vi "Window_plot.vi"() -> ()   [LabVIEW 2022 SP3]
doc: "This window has the capability to visualize and analyze the graphs of the stored signals from the Main_menu."
uses:
  <vilib>/Waveform/WDTOps.llb/WDT Get Waveform Subset DBL.vi
panel:
  in  "Slide Offset":i32(slide) scale=0.0..10.0
  in  "Select offset":string(combo)
  out "Waveform Graph":waveform(dbl)[](graph) caption="Waveform Graph 2"
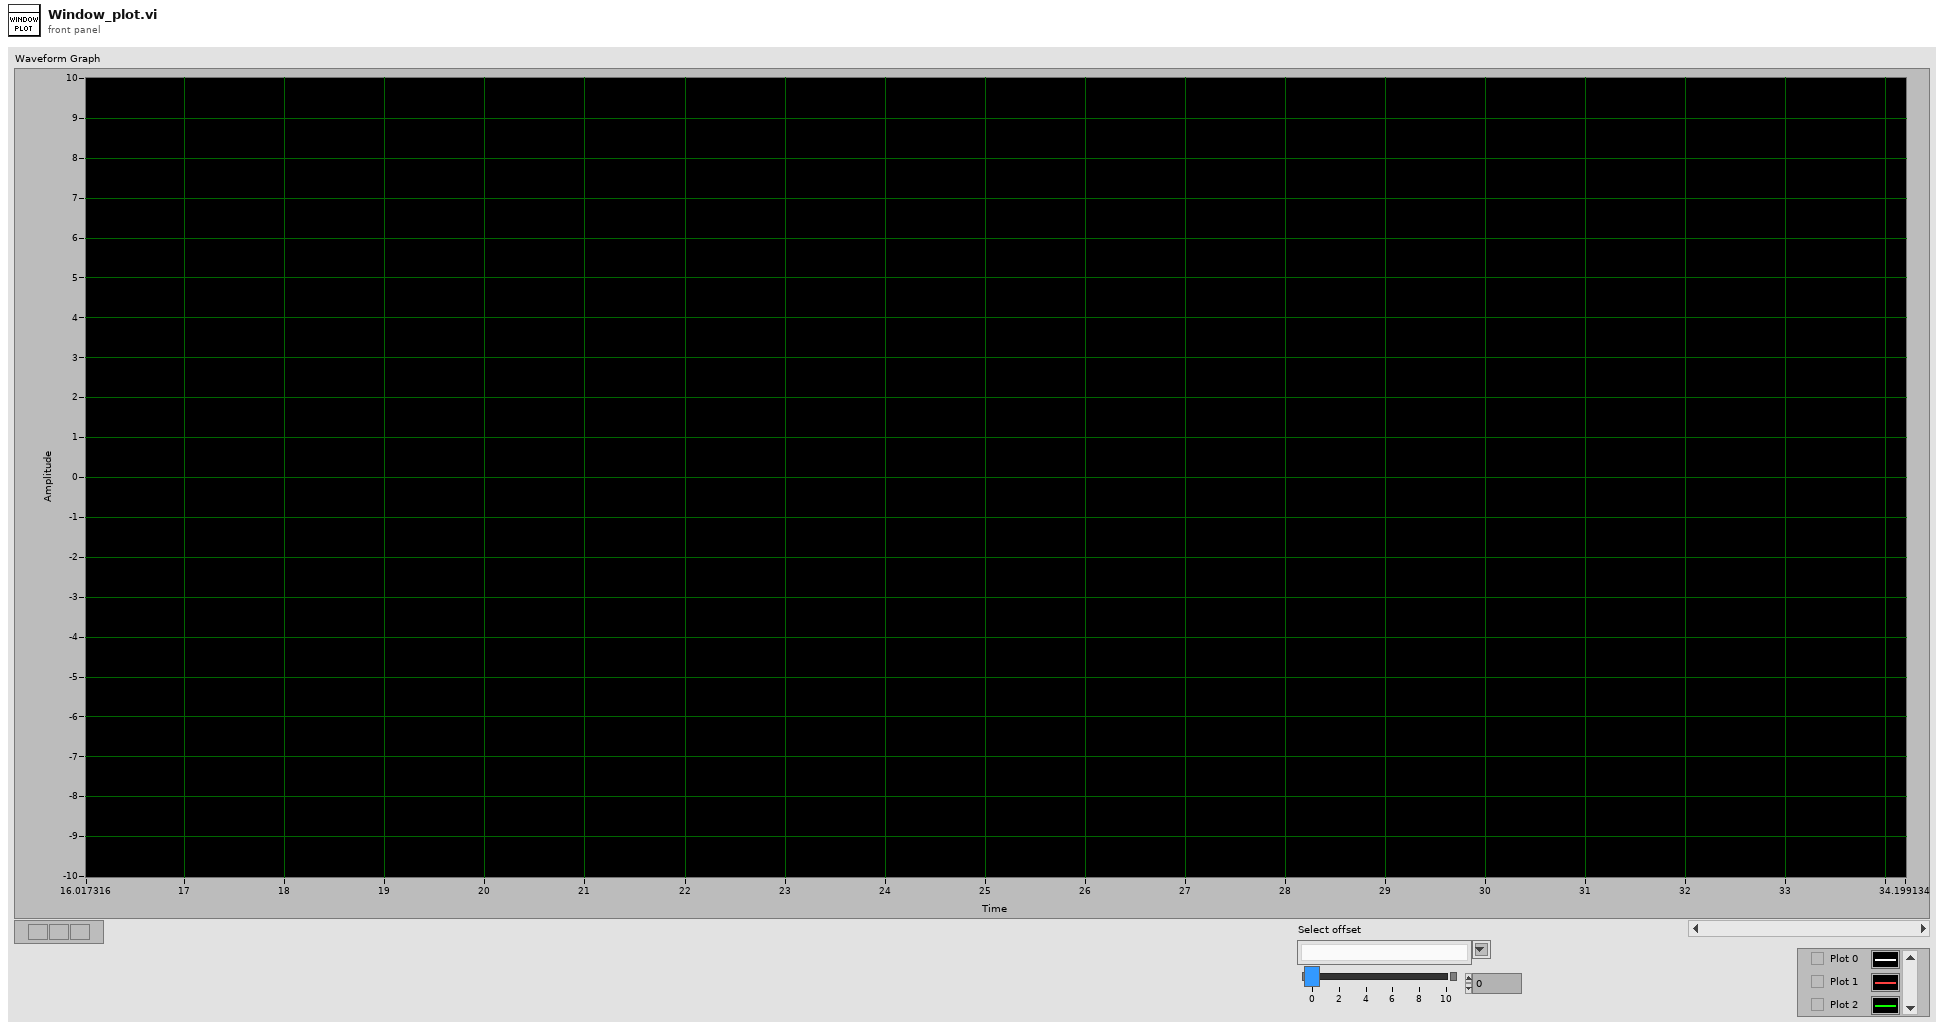
[diagram p1: front panel]
types:
  T1 = cluster{"Mode signal_Global":refnum<vi>, "Trace name":refnum<vi>, "Execution:State":refnum<vi>, "message":refnum<vi>, "Filename":refnum<vi>, "Closed w":refnum<vi>, "total \nrefresh time":refnum<vi>, "Mode signal_Global 2":string, "Filename 2":string, "Execution:State 2":enum32{"Bad", "Idle", "Run top level", "Running"}, "message 2":string, "Trace name 2":string, "total refresh time 2":i32, "refresh time 2":i32, "Continous":bool}
  T2 = cluster{"plot Names":string[], "Waveforms arrays":waveform(dbl)[], "signals_HW":string[][], "Waveforms arrays csv":waveform(dbl)[], "signals_csv":string[], "Signals_name":string[], "Mode_signal_conf":u8, "Request_plots_array":cluster{string, waveform(dbl)}[], "time out":i32, " global r time":u32, "Refresh time":u32, "Local Mode":enum32{"Resume", "Hold"}}
  T3 = enum32{"Invalid", "Standard", "Closed", "Hidden", "Minimized", "Maximized"}
  T4 = enum32{"Bad", "Idle", "Run top level", "Running"}
  T5 = cluster{"plot Names":string[], "Waveforms arrays":waveform(dbl)[], "signals_HW":string[][], "Waveforms arrays csv":waveform(dbl)[], "signals_csv":string[], "Signals_name":string[], "Mode_signal_conf":u8, "Request_plots_array":cluster{string, "Waveform":waveform(dbl)}[], "time out":i32, " global r time":u32, "Refresh time":u32, "Local Mode":enum32{"Resume", "Hold"}}
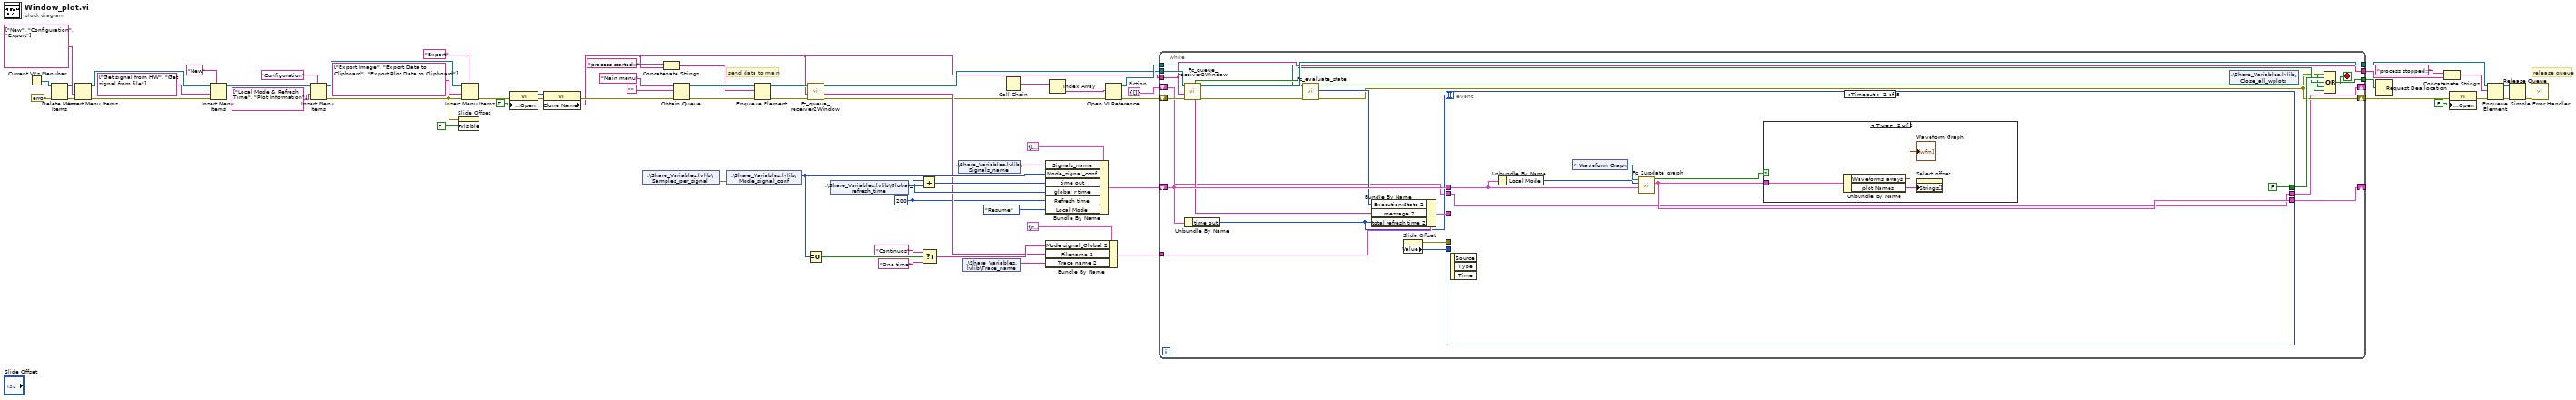
[diagram p0: block diagram]
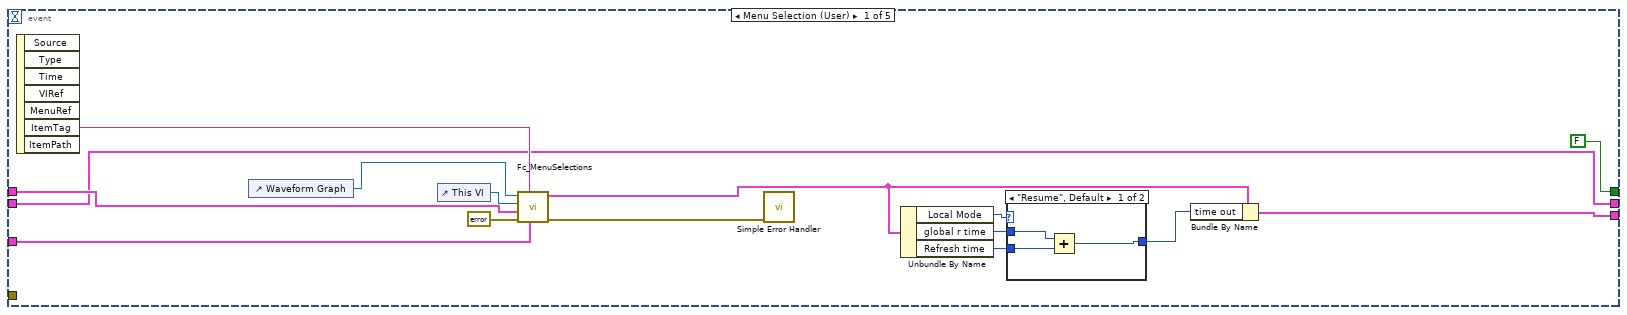
[diagram p2: hidden frame]
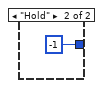
[diagram p3: hidden frame]
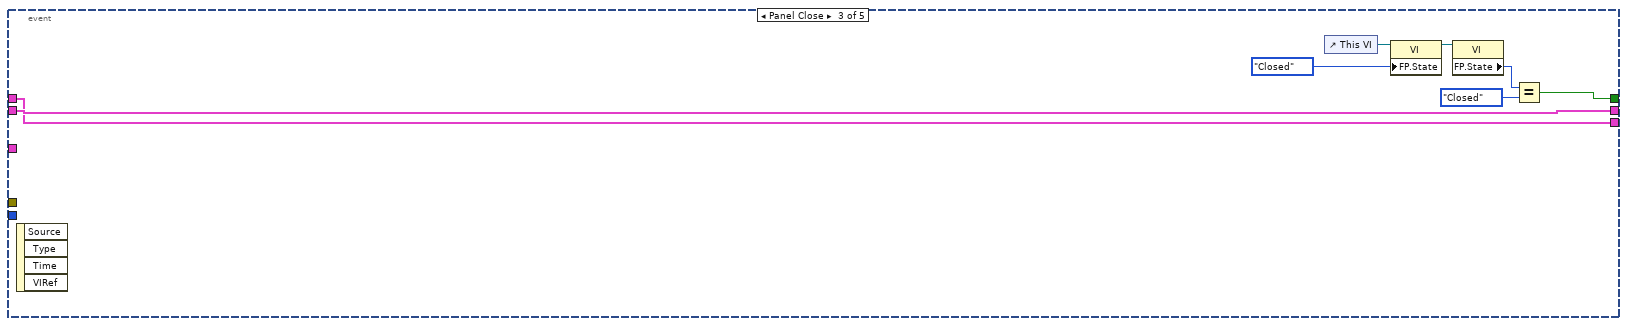
[diagram p5: hidden frame]
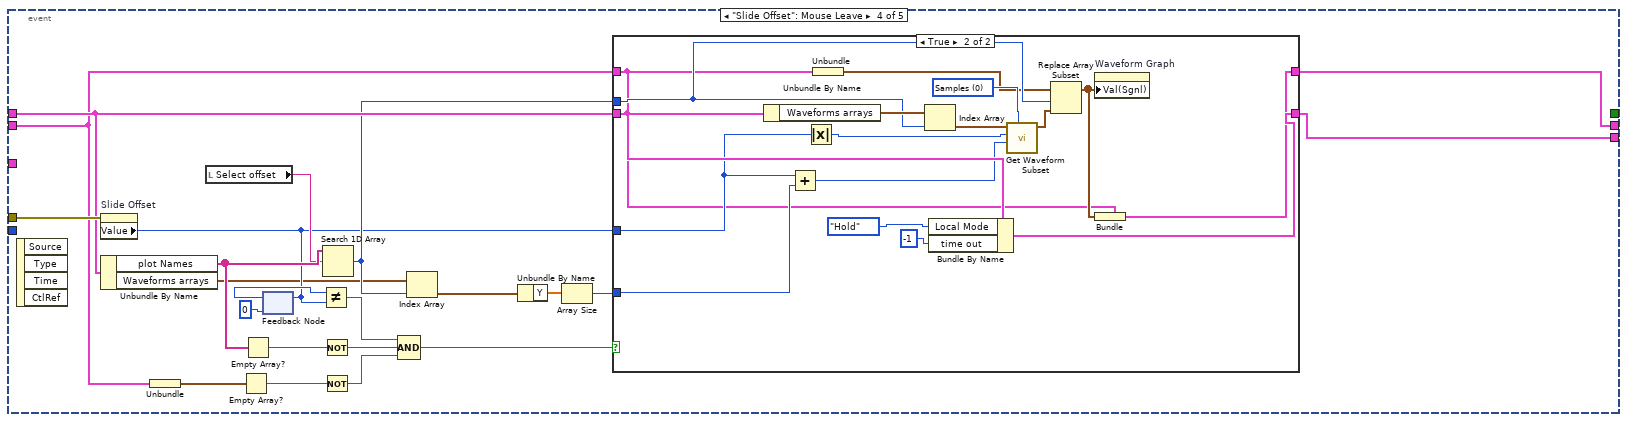
[diagram p6: hidden frame]
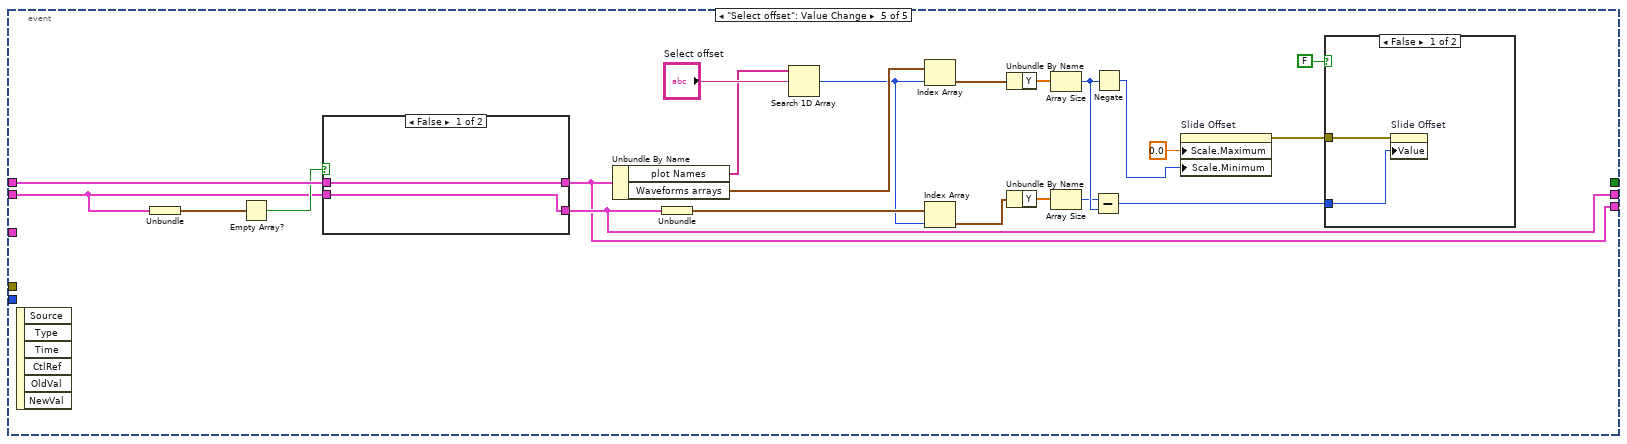
[diagram p8: hidden frame]
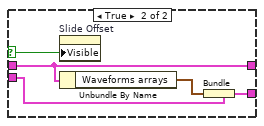
[diagram p10: hidden frame]
diagram:
  w5 = cluster{"Fiction Wavef":waveform(dbl)[]} {"Fiction Wavef"=[]}  # Fiction
  w30 = u32 200 ("Refresh time")
  # "send data to main"
  # "release queue"
  n1 = Current VI's Menubar() -> (w19:refnum<k9>)
  n2 = Delete Menu Items(6:errorcluster {"status"=FALSE, "code"=0, "source"=""} ("error in (no error)"), 9:w19) -> (0:w18:errorcluster, 3:w17:refnum<k9>)  [unwired: 2 in]
  n3 = Insert Menu Items(6:w18, 7:string[] ["New", "Configuration", "Export"], 9:w17) -> (0:w24:errorcluster, 3:w23:refnum<k9>)  [unwired: 3 in, 1 out]
  n4 = Insert Menu Items(5:"New", 6:w24, 7:string[] ["Get signal from HW", "Get signal from file"], 9:w23) -> (3:w12:refnum<k9>)  [unwired: 2 in, 2 out]
  n5 = Insert Menu Items(5:"Configuration" ("menu tag"), 7:string[] ["Local Mode & Refresh Time", "Plot Information"] ("item tags"), 9:w12) -> (0:w2:errorcluster, 3:w11:refnum<k9>)  [unwired: 3 in, 1 out]
  n6 = property on="Slide Offset" class="Slide (strict)"(error in=w2, "Visible"=FALSE) -> ()  [unwired: 1 in, 2 out]
  n7 = Insert Menu Items(5:"Export" ("menu tag"), 6:w2, 7:string[] ["Export Image", "Export Data to Clipboard", "Export Plot Data to Clipboard"], 9:w11) -> (0:w25:errorcluster)  [unwired: 2 in, 2 out]
  n8 = property class="VI"(error in=w25, "Front Panel.Open"=TRUE ("Front Panel Window:Open")) -> (reference out=w50:refnum<vi>, error out=w60:errorcluster)  [unwired: 1 in]
  n9 = property class="VI"(reference=w50, error in=w60) -> (error out=w43:errorcluster, "Clone Name"=w33:string)  [unwired: 1 out]
  n10 = shared-variable ".\\Share_Variables.lvlib\\Samples_per_signal"() -> (error out=w3:errorcluster)  [unwired: 1 in, 1 out]
  n11 = Concatenate Strings("process started::" ("name (unnamed)"), w33) -> (w61:string)
  n12 = Obtain Queue(name (unnamed)="Main menu", element data type="", error in (no error)=w43) -> (queue out=w63:refnum<queue>, error out=w62:errorcluster)  [unwired: 2 in, 1 out]
  n13 = shared-variable ".\\Share_Variables.lvlib\\Mode_signal_conf"(error in=w3) -> (w44:u8)  [unwired: 1 out]
  n14 = Enqueue Element(queue=w63, element=w61, error in (no error)=w62) -> (queue out=w36:refnum<queue>, error out=w34:errorcluster)  [unwired: 1 in, 1 out]
  n15 = Equal To 0?(x=w44) -> (x = 0?=w8:bool)
  n16 = call "Fc_queue_receiver2Window.vi"("error in (no error)"=w34, "Clone Name"=w33, "Queue in"=w36) -> ("error out"=w6:errorcluster, "Filename"=w31:string, "Queue out"=w35:refnum<queue>)  [unwired: 4 in, 2 out]
  n17 = shared-variable ".\\Share_Variables.lvlib\\Global_refresh_time"() -> (w39:u16)  [unwired: 1 in, 1 out]
  n18 = Add(x=w30, y=w39) -> (x+y=w40:u32)
  n19 = Select(t="Continuos", s=w8, f="One time") -> (s? t:f=w32:string)
  n20 = shared-variable ".\\Share_Variables.lvlib\\Signals_name"() -> (w45:string[])  [unwired: 1 in, 1 out]
  n21 = shared-variable ".\\Share_Variables.lvlib\\Trace_name"() -> (w29:string)  [unwired: 1 in, 1 out]
  n22 = Call Chain() -> (call chain=w49:string[])
  n23 = Bundle By Name(cluster=T2 {"plot Names"=[], "Waveforms arrays"=[], "signals_HW"=[], "Waveforms arrays csv"=[], "signals_csv"=[], "Signals_name"=[], "Mode_signal_conf"=0, "Request_plots_array"=[], "time out"=300, " global r time"=0, "Refresh time"=0, "Local Mode"=enum."Resume"}, "Signals_name"=w45, "Mode_signal_conf"=w44, "time out"=w40, "global r time"=w39, "Refresh time"=w30, "Local Mode"=enum32{"Resume", "Hold"}."Resume") -> (w46:T2)
  n24 = Bundle By Name(cluster=T1 {"Mode signal_Global"=refnum, "Trace name"=refnum, "Execution:State"=refnum, "message"=refnum, "Filename"=refnum, "Closed w"=refnum, "total \nrefresh time"=refnum, "Mode signal_Global 2"="", "Filename 2"="", "Execution:State 2"=enum."Idle", "message 2"="", "Trace name 2"="", "total refresh time 2"=0, "refresh time 2"=0, "Continous"=TRUE}, "Mode signal_Global 2"=w32, "Filename 2"=w31, "Trace name 2"=w29) -> (w38:T1)
  n25 = Index Array(array=w49) -> (element=w48:string)  [unwired: 1 in]
  n26 = Open VI Reference(vi path=w48, error in (no error)=w6) -> (vi reference=w47:refnum<vi>, error out=w27:errorcluster)  [unwired: 4 in]
  n27 = while {
    tunnel: w35 -> [w89]
    tunnel: [w88] -> w59
    shift-right: [w72] -> w54
    shift-left: w27 -> [w78]
    tunnel: [w83] -> w52
    tunnel: w47 -> [w81]
    tunnel: w33 -> [w83]
    shift-right: [w84] -> _
    shift-left: w46 -> [w82]
    tunnel: [w80] -> w42
    tunnel: w38 -> [w77]
    shift-right: [w68] -> _
    shift-left: w5 -> [w69]
    stop <- w80 stop-if-true
    n28 = call "Fc_queue_receiver2Window.vi"("error in (no error)"=w78, "Clone Name"=w83, "Queue in"=w89) -> ("error out"=w67:errorcluster, "Queue out"=w88:refnum<queue>, "message"=w74:string, "Stop"=w86:bool)  [unwired: 4 in, 1 out]
    n29 = Unbundle By Name(w82) -> ("time out"=w73:i32)
    n30 = call "Fc_evaluate_state.vi"("error in (no error)"=w67, "VI in"=w81) -> ("error out"=w72:errorcluster, "Exec.State"=w76:T4, "Status out"=w79:bool)  [unwired: 7 in]
    n31 = Bundle By Name(cluster=w77, "Execution:State 2"=w76, "message 2"=w74, "total refresh time 2"=w73) -> (w75:T1)
    n32 = property on="Slide Offset" class="Slide (strict)"() -> (error out=w71:errorcluster, "Value"=w70:i32)  [unwired: 2 in, 1 out]
    n33 = event shown="[1] Timeout" {
      selector: _ -> [_ _ _ _ _]
      dyn-events: _ -> [_ _ _ _ _]
      timeout: w73 -> [_ _ _ _ _]
      tunnel: [FALSE FALSE w124 _ _] -> w87
      tunnel: [w91 w110 w119 w144 w170] -> w84
      tunnel: w82 -> [w96 w112 w119 w145 w184]
      tunnel: w75 -> [w98 _ _ _ _]
      tunnel: w71 -> [_ _ _ w148 _]
      tunnel: w70 -> [_ _ _ _ _]
      tunnel: w69 -> [w90 w109 w120 w139 w182]
      tunnel: [w90 w109 w120 w138 w178] -> w68
      event Menu Selection (User) {
        n34 = event-data() -> ("ItemTag"=w104:string)  [unwired: 1 in, 6 out]
        n35 = control-ref of="Waveform Graph"() -> (w100:refnum<vi>)
        n36 = control-ref of="This VI"() -> (w99:refnum<vi>)
        n37 = call "Fc_MenuSelections.vi"("Cluster References"=w98, "ItemTag"=w104, "error in (no error)"=errorcluster {"status"=FALSE, "code"=0, "source"=""}, "Cluster in"=w96, "VI caller"=w99, "WaveformGraph in"=w100) -> ("error out"=w102:errorcluster, "Cluster out"=w92:T5)  [unwired: 4 in]
        n38 = call <vilib>:"Simple Error Handler.vi"("error in (no error)"=w102) -> ()  [unwired: 4 in, 5 out]
        n39 = Unbundle By Name(w92) -> ("Local Mode"=w95:enum32{"Resume", "Hold"}, "global r time"=w94:u32, "Refresh time"=w93:u32)
        n40 = case shown="\"Resume\", Default" w95 {
          tunnel: [w105 -1 ("time out")] -> w97
          tunnel: w94 -> [w107 _]
          tunnel: w93 -> [w106 _]
          frame "Resume", Default {
            n41 = Add(x=w107, y=w106) -> (x+y=w105:u32)
          }
          frame "Hold" {
          }
        }
        n42 = Bundle By Name(cluster=w92, "time out"=w97) -> (w91:T5)
      }
      event Timeout {
        n43 = event-data() -> ()  [unwired: 1 in, 3 out]
        n44 = Unbundle By Name(w112) -> ("Local Mode"=w111:enum32{"Resume", "Hold"})
        n45 = control-ref of="Waveform Graph"() -> (w113:refnum<vi>)
        n46 = call "Fc_2update_graph.vi"("Cluster in"=w112, "Local Mode"=w111, "WaveformGraph in"=w113) -> ("Cluster in 2"=w110:T5, "Update Waveform Graph"=w114:bool)  [unwired: 7 in]
        n47 = case shown="True" w114 {
          tunnel: w110 -> [_ w117]
          frame False {
          }
          frame True {
            n48 = Unbundle By Name(w117) -> ("Waveforms arrays"=→"Waveform Graph":waveform(dbl)[], "plot Names"=w116:string[])
            n49 = property on="Select offset" class="CmbBox"("Strings[]"=w116) -> ()  [unwired: 2 in, 2 out]
          }
        }
      }
      event Panel Close {
        n50 = event-data() -> ()  [unwired: 1 in, 4 out]
        n51 = control-ref of="This VI"() -> (w123:refnum<vi>)
        n52 = property class="VI"(reference=w123, "FP.State"=T3."Closed" ("Front Panel Window:State")) -> (reference out=w121:refnum<vi>)  [unwired: 1 in, 1 out]
        n53 = property class="VI"(reference=w121) -> ("FP.State"=w125:T3)  [unwired: 1 in, 2 out]
        n54 = Equal?(x=w125, y=T3."Closed" ("Front Panel Window:State")) -> (x = y?=w124:bool)
      }
      event "Slide Offset": Mouse Leave {
        n55 = event-data() -> ()  [unwired: 1 in, 4 out]
        n56 = property on="Slide Offset" class="Slide (strict)"(error in=w148) -> ("Value"=w130:i32)  [unwired: 1 in, 2 out]
        n57 = Unbundle By Name(w145) -> ("plot Names"=w146:string[], "Waveforms arrays"=w127:waveform(dbl)[])
        n58 = Unbundle(w139) -> ("Fiction Wavef"=w136:waveform(dbl)[])
        n59 = local read "Select offset"() -> (w137:string)
        n60 = Empty Array?(array=w136) -> (empty?=w133:bool)
        n61 = Empty Array?(array=w146) -> (empty?=w135:bool)
        n62 = feedback #1(0 ("Value")) -> (w131:i32)
        n63 = feedback-in #1(w130) -> ()
        n64 = Not Equal?(x=w131, y=w130) -> (x != y?=w128:bool)
        n65 = Not(x=w135) -> (.not. x?=w134:bool)
        n66 = Not(x=w133) -> (.not. x?=w132:bool)
        n67 = Search 1D Array(1D array=w146, element=w137) -> (index of element=w143:i32)  [unwired: 1 in]
        n68 = Compound Arithmetic op=AND(w128, w134, w132) -> (w147:bool)
        n69 = Index Array(array=w127, index=w143) -> (element=w142:waveform(dbl))
        n70 = Unbundle By Name(w142) -> ("Y"=w141:dbl[])
        n71 = Array Size(array=w141) -> (size(s)=w140:i32)
        n72 = case shown="True" w147 {
          tunnel: w145 -> [w150 w159]
          tunnel: w143 -> [_ w160]
          tunnel: w130 -> [_ w154]
          tunnel: [w150 w163] -> w144
          tunnel: w140 -> [_ w158]
          tunnel: w139 -> [w149 w152]
          tunnel: [w149 w156] -> w138
          frame False {
          }
          frame True {
            w167 = u16 0 items=["Samples", "Relative Time"] ("start/duration format")
            n73 = Unbundle By Name(w159) -> ("Waveforms arrays"=w165:waveform(dbl)[])
            n74 = Add(x=w154, y=w158) -> (x+y=w153:i32)
            n75 = Absolute Value(x=w154) -> (abs(x)=w155:i32)
            n76 = Unbundle(w152) -> ("Fiction Wavef"=w151:waveform(dbl)[])
            n77 = Index Array(array=w165, index=w160) -> (element=w166:waveform(dbl))
            n78 = Bundle By Name(cluster=w159, "Local Mode"=enum32{"Resume", "Hold"}."Hold", "time out"=-1) -> (w163:T2)
            n79 = call-poly <vilib>:"Get Waveform Subset.vi"("start/duration format"=w167, "duration"=w153, "start samples/time"=w155, "waveform in"=w166) -> ("waveform out"=w164:waveform(dbl))  [unwired: 2 in, 3 out]
            n80 = Replace Array Subset(array=w151, new element=w164, index=w160) -> (w157:waveform(dbl)[])
            n81 = property on="Waveform Graph" class="WFGraph (strict)"("Val(Sgnl)"=w157) -> ()  [unwired: 2 in, 2 out]
            n82 = Bundle(cluster=w152, "Fiction Wavef"=w157) -> (w156:cluster{"Fiction Wavef":waveform(dbl)[]})
          }
        }
      }
      event "Select offset": Value Change {
        n83 = event-data() -> ()  [unwired: 1 in, 6 out]
        n84 = Unbundle(w182) -> ("Fiction Wavef"=w169:waveform(dbl)[])
        n85 = Empty Array?(array=w169) -> (empty?=w183:bool)
        n86 = case shown="False" w183 {
          selector: w183 -> [_ w194]
          tunnel: w184 -> [w192 w195]
          tunnel: w182 -> [w193 w197]
          tunnel: [w193 w196] -> w178
          tunnel: [w192 w195] -> w170
          frame False {
          }
          frame True {
            n87 = property on="Slide Offset" class="Slide (strict)"("Visible"=w194) -> ()  [unwired: 2 in, 2 out]
            n88 = Unbundle By Name(w195) -> ("Waveforms arrays"=w198:waveform(dbl)[])
            n89 = Bundle(cluster=w197, "Fiction Wavef"=w198) -> (w196:cluster{"Fiction Wavef":waveform(dbl)[]})
          }
        }
        n90 = Unbundle By Name(w170) -> ("plot Names"=w188:string[], "Waveforms arrays"=w187:waveform(dbl)[])
        n91 = Unbundle(w178) -> ("Fiction Wavef"=w177:waveform(dbl)[])
        n92 = Search 1D Array(1D array=w188, element="Select offset") -> (index of element=w176:i32)  [unwired: 1 in]
        n93 = Index Array(array=w187, index=w176) -> (element=w186:waveform(dbl))
        n94 = Index Array(array=w177, index=w176) -> (element=w175:waveform(dbl))
        n95 = Unbundle By Name(w186) -> ("Y"=w185:dbl[])
        n96 = Unbundle By Name(w175) -> ("Y"=w174:dbl[])
        n97 = Array Size(array=w185) -> (size(s)=w181:i32)
        n98 = Array Size(array=w174) -> (size(s)=w173:i32)
        n99 = Subtract(x=w173, y=w181) -> (x-y=w172:i32)
        n100 = Negate(x=w181) -> (-x=w180:i32)
        n101 = property on="Slide Offset" class="Slide (strict)"("Scale.Maximum"=0.0 ("Scale.Range:Maximum"), "Scale.Minimum"=w180) -> (error out=w171:errorcluster)  [unwired: 2 in, 1 out]
        n102 = case shown="False" FALSE {
          tunnel: w172 -> [w191 _]
          tunnel: w171 -> [w190 _]
          frame False {
            n103 = property on="Slide Offset" class="Slide (strict)"(error in=w190, "Value"=w191) -> ()  [unwired: 1 in, 2 out]
          }
          frame True {
          }
        }
      }
    }
    n104 = shared-variable ".\\Share_Variables.lvlib\\Close_all_wplots"() -> (w85:bool)  [unwired: 1 in, 1 out]
    n105 = Compound Arithmetic op=OR(w72, w87, w86, w85, w79) -> (w80:bool)
  }
  n106 = Request Deallocation(w42) -> ()
  n107 = Concatenate Strings("process stopped::" ("string"), w52) -> (w51:string)
  n108 = property class="VI"(error in=w54, "Front Panel.Open"=FALSE ("Front Panel Window:Open")) -> (error out=w56:errorcluster)  [unwired: 1 in, 1 out]
  n109 = Enqueue Element(queue=w59, element=w51, error in (no error)=w56) -> (queue out=w58:refnum<queue>, error out=w57:errorcluster)  [unwired: 1 in, 1 out]
  n110 = Release Queue(queue=w58, error in (no error)=w57) -> (error out=w28:errorcluster)  [unwired: 1 in, 2 out]
  n111 = call <vilib>:"Simple Error Handler.vi"("error in (no error)"=w28) -> ()  [unwired: 4 in, 5 out]
